vi "ReteachTravPosition.vi"(3 "Mode":T1, 5 "Traverse line In":T2 {"Carrier_2 Q (l/min)" format="%#.2f"; "Row Duration (mins)" format="%#.1f"; "Row No" min=0; "Trace Gas Concentration (%)" min=0.0 format="%#_4f"; "Carrier_1 Q (l/min)" format="%#.2f"; "Tunnel Speed" format="%#.2f"; "Start X" format="%#.2f"; "Start Y" format="%#.2f"; "Start Z" format="%#.2f"; "End X" format="%#.2f"; "End Y" format="%#.2f"; "End Z" format="%#.2f"; "Averaging time (min)" min=0.0 format="%#.2f"}) -> (0 "Error Message":string, 1 "Status":T5, 2 "Traverse line Out":T2 {"Carrier_2 Q (l/min)" format="%#.2f"; "Row Duration (mins)" format="%#.1f"; "Row No" min=0; "Trace Gas Concentration (%)" min=0.0 format="%#_4f"; "Carrier_1 Q (l/min)" format="%#.2f"; "Tunnel Speed" format="%#.2f"; "Start X" format="%#.2f"; "Start Y" format="%#.2f"; "Start Z" format="%#.2f"; "End X" format="%#.2f"; "End Y" format="%#.2f"; "End Z" format="%#.2f"; "Averaging time (min)" min=0.0 format="%#.2f"})   [LabVIEW 2015]
uses:
  Gen Trav/Multi_Run_Status.ctl
  Gen Trav/Trav_mode.ctl
  Gen Trav/Spacing.ctl
  Controls/Multi_run_mode.ctl
  Gen Trav/Traverse_cluster.ctl
  Controls/User_Specific_mode.ctl
panel:
  # "X           Y            Z"
  # "Start"
  # "End"
  # "X           Y            Z"
  # "Start"
  # "End"
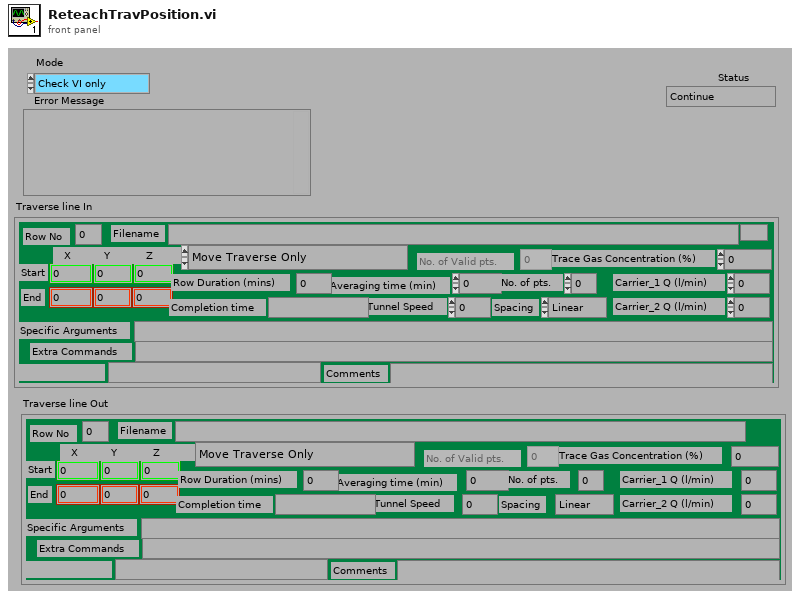
[diagram p1: front panel]
types:
  T1 = typedef "User_Specific_mode.ctl" = enum16{"Check VI only", "Run VI"}
  T2 = typedef "Traverse_cluster.ctl" = cluster{"Start X":sgl, "Start Y":sgl, "Start Z":sgl, "End X":sgl, "End Y":sgl, "End Z":sgl, "No. of pts.":i32, "Spacing":T3, "Filename":path, "Tunnel Speed":dbl, "Averaging time (min)":dbl, "Extra Commands":string, "Carrier_1 Q (l/min)":dbl, "Carrier_2 Q (l/min)":dbl, "Trace Gas Concentration (%)":dbl, "Specific Arguments":string, "Comments":string, "Row No":i32, "Row Type Selector":T4, "Completion time":string, "Row Duration (mins)":dbl, "No. of Valid pts.":i32, "Meas Setup File":string}
  T3 = typedef "Spacing.ctl" = enum16{"Linear", "Log", "Gauss", "Specified", "N/A"}
  T4 = typedef "Multi_run_mode.ctl" = enum16{"Move Traverse Only", "Set Tunnel Speed Only", "Set Source Only", "Set Measurement Conditions", "Single Measurement", "Vertical Profile", "Lateral Profile", "Longitudinal Profile", "Explore Volume", "Multi-Axis Profile", "Auto Calibrate", "Meas Fast FID Bkgnd", "Check Beam Power", "Scanning Valve Measurement", "Run VI Named:", "Set ADAM Ch", "Wait (minutes)", "Send Message", "Synchronize With:", "Fall Back to this Row", "Turn Off Row Repeating", "Blank Row", "Traverse 3D Volume"}
  T5 = typedef "Multi_Run_Status.ctl" = enum16{"Continue", "Jump to Next Point", "Jump to Next Row", "Jump To Fall Back", "Terminate Run"}
  T6 = typedef "Trav_mode.ctl" = enum16{"Move traverse", "Read traverse position", "Teach Position"}
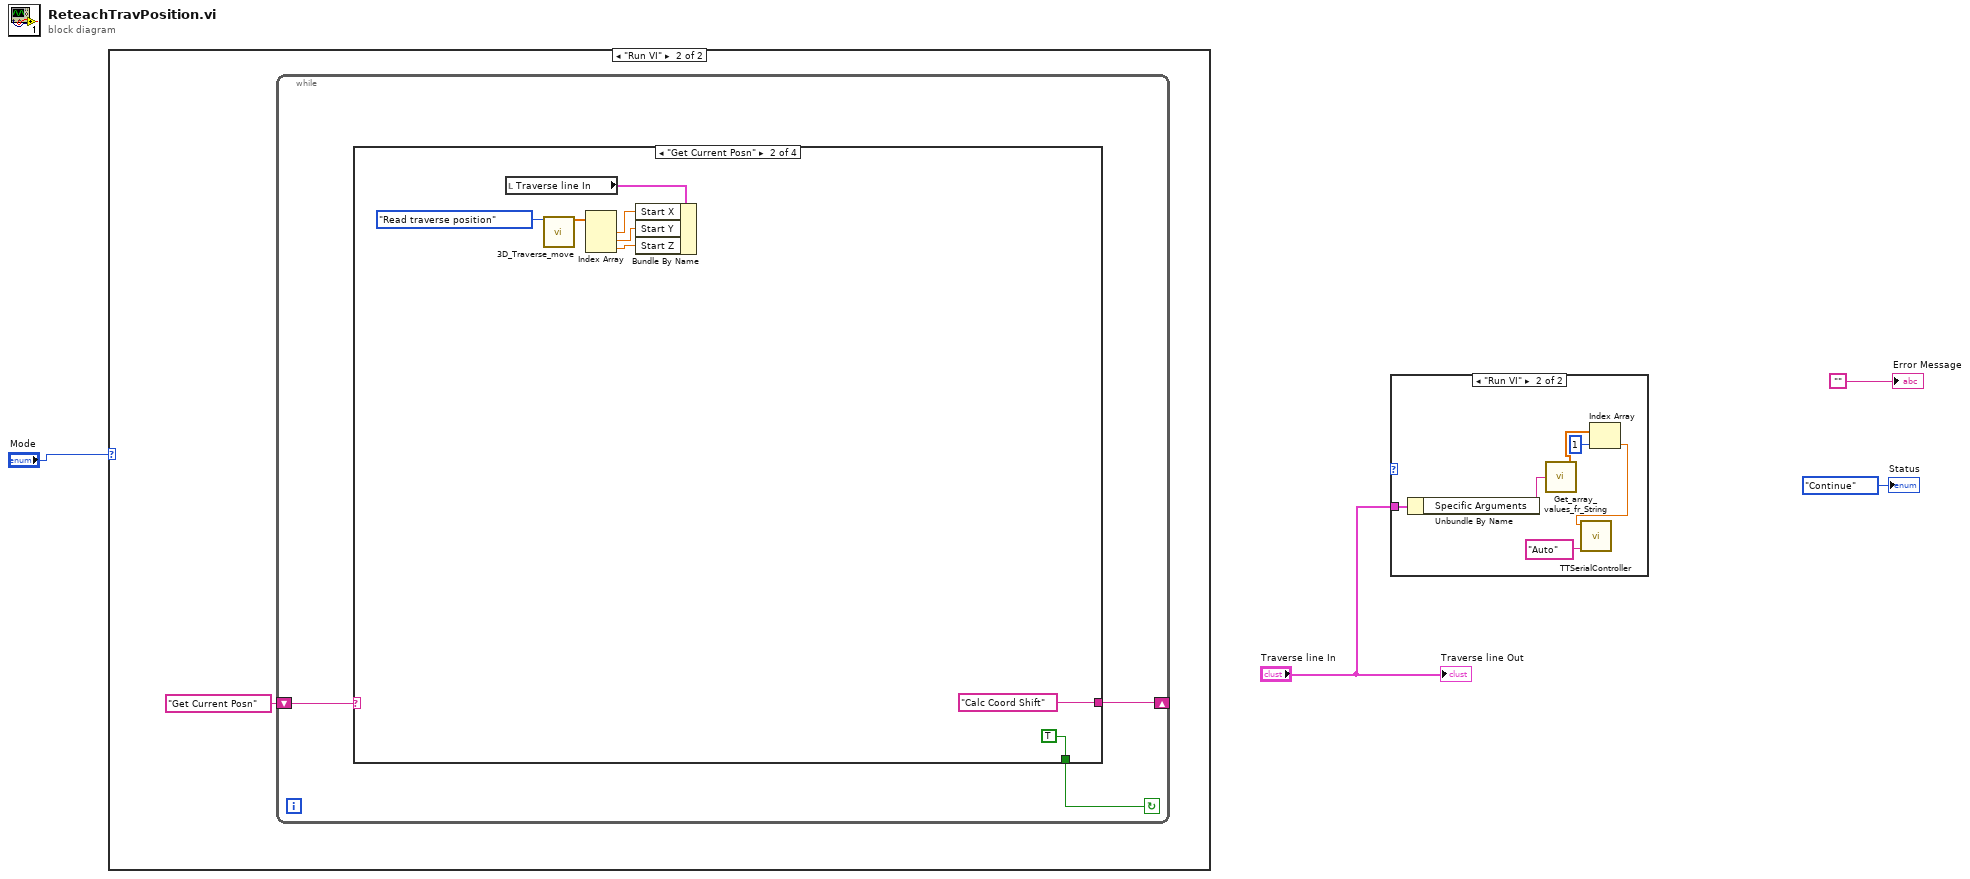
[diagram p0: block diagram]
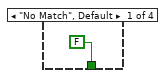
[diagram p3: hidden frame]
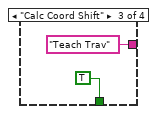
[diagram p4: hidden frame]
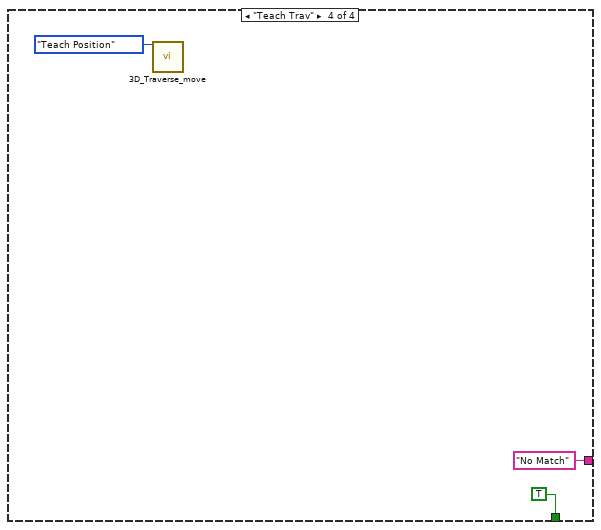
[diagram p5: hidden frame]
diagram:
  n1 = case shown="\"Run VI\"" "Mode" {
    frame "Check VI only", Default {
    }
    frame "Run VI" {
      n2 = while {
        shift-right: [w7] -> _
        shift-left: "Get Current Posn" -> [w8]
        stop <- w6 continue-if-true
        n3 = case shown="\"Get Current Posn\"" w8 {
          tunnel: [_ "Calc Coord Shift" "Teach Trav" "No Match"] -> w7
          tunnel: [FALSE TRUE TRUE TRUE] -> w6
          frame "No Match", Default {
          }
          frame "Get Current Posn" {
            n4 = local read "Traverse line In"() -> (w14:T2)
            n5 = call "3D_Traverse_move.vi"("Mode"=Trav_mode."Read traverse position") -> ("Trav Position achieved"=w13:sgl[])  [unwired: 16 in, 2 out]
            n6 = Index Array(array=w13) -> (element #1=w12:sgl, element #2=w11:sgl, element #3=w10:sgl)  [unwired: 3 in]
            n7 = Bundle By Name(cluster=w14, "Start X"=w12, "Start Y"=w11, "Start Z"=w10) -> ()  [unwired: 1 out]
          }
          frame "Calc Coord Shift" {
          }
          frame "Teach Trav" {
            n8 = call "3D_Traverse_move.vi"("Mode"=Trav_mode."Teach Position") -> ()  [unwired: 16 in, 3 out]
          }
        }
      }
    }
  }
  n9 = case shown="\"Run VI\"" {
    selector: _ -> [_ _]
    tunnel: "Traverse line In" -> [_ w28]
    frame "Check VI only", Default {
    }
    frame "Run VI" {
      n10 = Unbundle By Name(w28) -> ("Specific Arguments"=w26:string)
      n11 = call "Get_array_values_fr_String.vi"("String Value"=w26) -> ("Numeric Array"=w24:dbl[])  [unwired: 1 out]
      n12 = Index Array(array=w24, index=1 ("Index")) -> (element=w23:dbl)
      n13 = call "TTSerialController.vi"("Mode"="Auto", "RequestedAzimuth"=w23) -> ()  [unwired: 9 in]
    }
  }
  "Status" <- Multi_Run_Status."Continue" ("Status")
  "Error Message" <- "" ("Error Message")
  "Traverse line Out" <- "Traverse line In"
